vi "Parse Data Frame.vi"(0 "VISA Session In":refnum<visa-resource-name>="Alicat", 5 "Unit ID (A)":string="A", 7 "Data Frame Input":string, 9 "Data Frame Format In":T1, 11 "error in":errorcluster, 13 "Offset (2 if polling, 0 if streaming)":u32=2) -> (1 "Range Exceeded":bool, 3 "Error/Overrange/Unknown String":string, 4 "VISA Session Out":refnum<visa-resource-name>, 6 "Data Cluster":T2, 10 "Data Frame Format Out":T1, 12 "Error Present":bool, 14 "Unknown Dataframe Info":bool, 15 "error out":errorcluster)   [LabVIEW 2016]
doc: "Parses data string obtained from an Alicat device according to data flag inputs, and if none are present the device will query the data flags (adding a considerable amount of time to the VI's execution). Outputs cluster of data, retrieved/used data flags, and error/overrange/unknown indicators and strings."
uses:
  <vilib>/Utility/error.llb/whitespace.ctl
panel:
  # "Totalizer Timer"
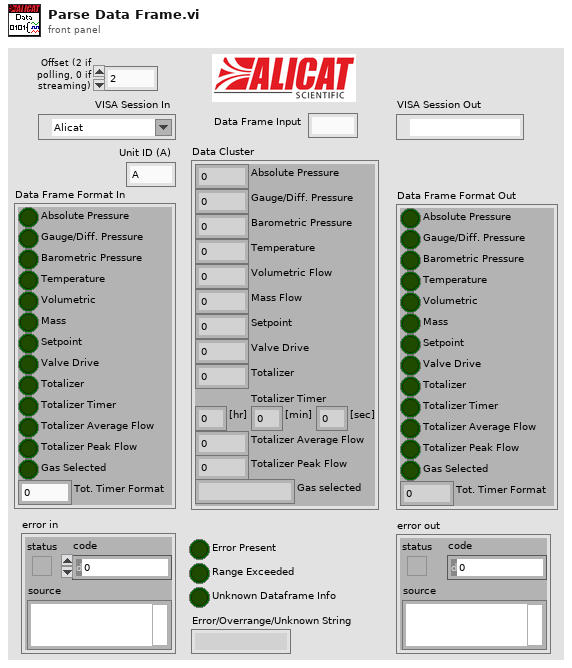
[diagram p1: front panel]
types:
  T1 = cluster{"Absolute Pressure":bool, "Gauge/Diff. Pressure":bool, "Barometric Pressure":bool, "Temperature":bool, "Volumetric":bool, "Mass":bool, "Setpoint":bool, "Valve Drive":bool, "Totalizer":bool, "Totalizer Timer":bool, "Totalizer Average Flow":bool, "Totalizer Peak Flow":bool, "Gas Selected":bool, "Tot. Timer Format":u16}
  T2 = cluster{"Absolute Pressure":dbl, "Gauge/Diff. Pressure":dbl, "Barometric Pressure":dbl, "Temperature":dbl, "Volumetric Flow":dbl, "Mass Flow":dbl, "Setpoint":dbl, "Valve Drive":dbl, "Totalizer":dbl, "[hr]":dbl, "[min]":dbl, "[sec]":dbl, "Totalizer Average Flow":dbl, "Totalizer Peak Flow":dbl, "Gas selected":string}
  T3 = cluster{"Absolute Pressure":dbl, "Gauge/Diff. Pressure":dbl, "Barometric Pressure":dbl, "Temperature":dbl, "Volumetric":dbl, "Mass":dbl, "Setpoint":dbl, "Valve Drive":dbl, "Totalizer":dbl, "[hr]":dbl, "[min]":dbl, "[sec]":dbl, "Totalizer Average Flow":dbl, "Totalizer Peak Flow":dbl, "Gas selected":string}
  T4 = typedef "whitespace.ctl" = u16
  T5 = cluster{"Absolute Pressure":bool, "Gauge/Diff. Pressure":bool, "Barometric Pressure":bool, "Temperature":bool, "Volumetric":bool, "Mass":bool, "Setpoint":bool, "Valve Drive":bool, "Totalizer":bool, "Totalizer Timer":bool, "Totalizer Average Flow":bool, "Totalizer Peak Flow":bool, "Gas Selected":bool}
  T6 = cluster{"[0]":dbl, "[1]":dbl, "[2]":dbl, "[3]":dbl, "[4]":dbl, "[5]":dbl, "[6]":dbl, "[7]":dbl, "[8]":dbl, "[9]":dbl, "[10]":dbl, "[11]":dbl}
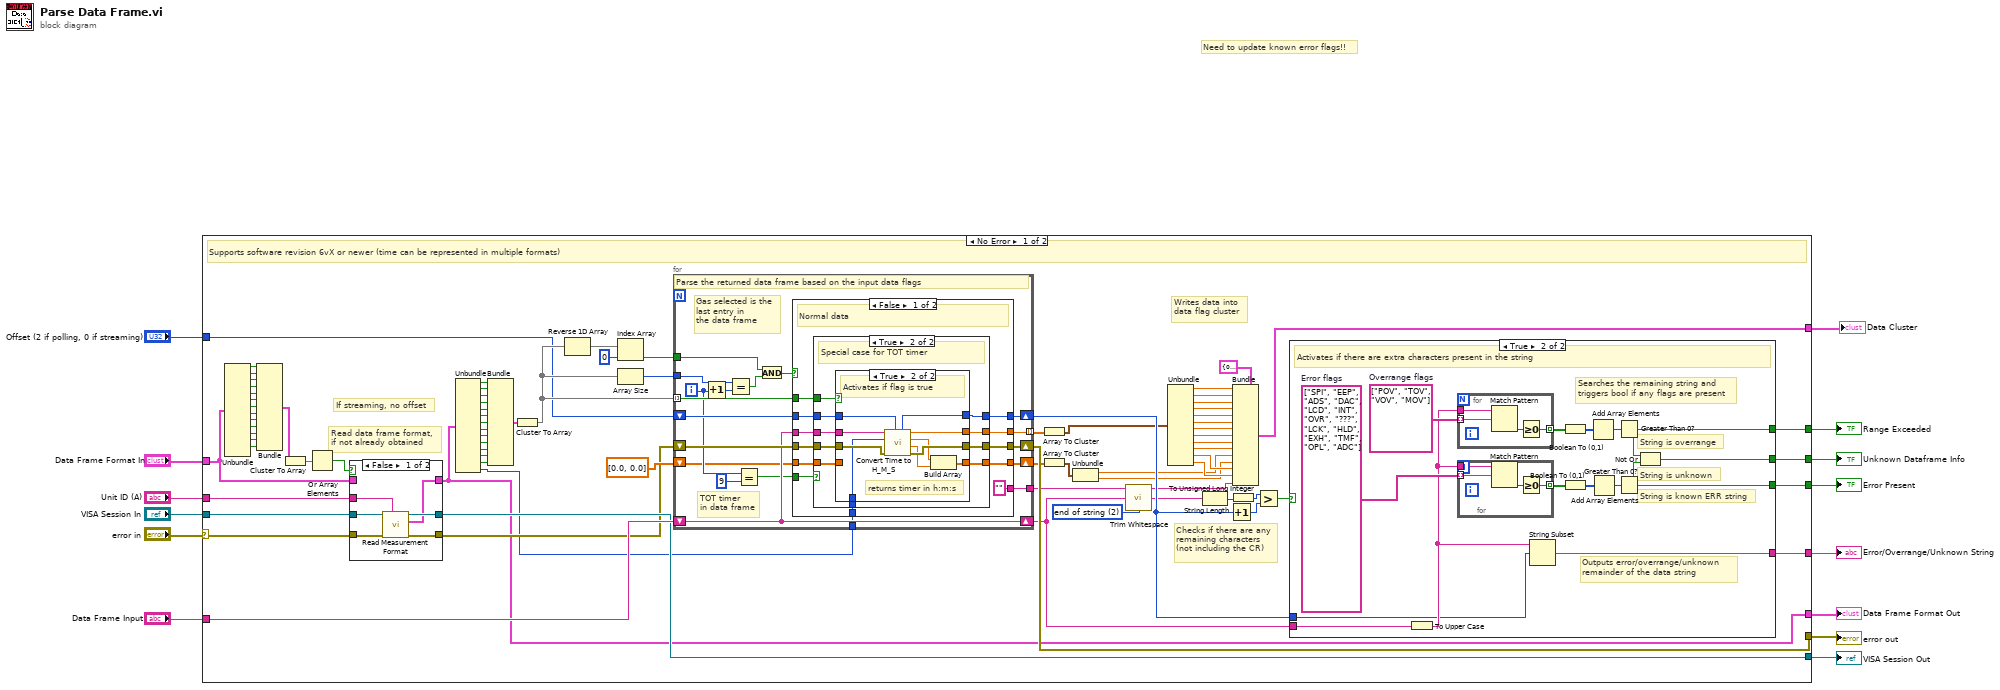
[diagram p0: block diagram]
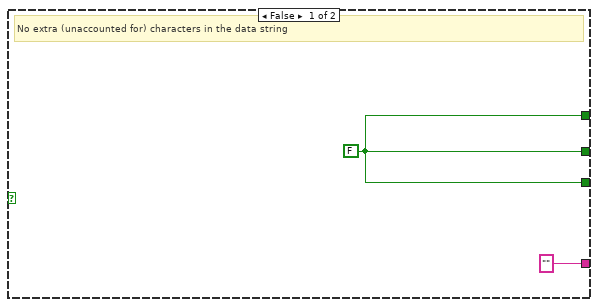
[diagram p2: hidden frame]
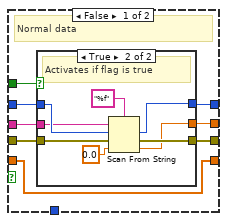
[diagram p3: hidden frame]
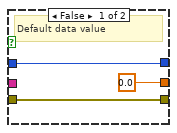
[diagram p4: hidden frame]
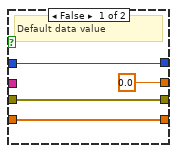
[diagram p5: hidden frame]
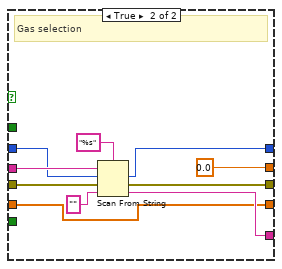
[diagram p6: hidden frame]
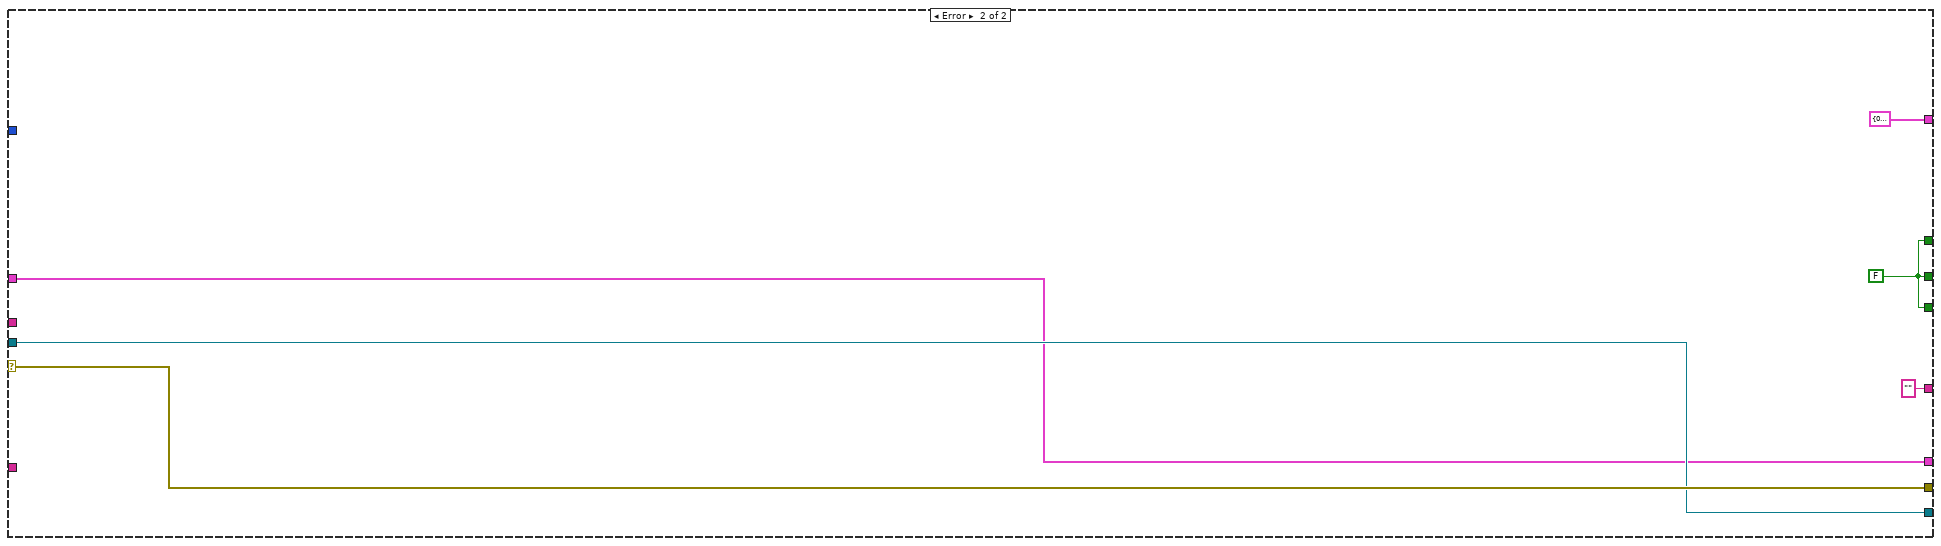
[diagram p8: hidden frame]
diagram:
  # "Need to update known error flags!!"
  n1 = case shown="No Error" "error in" {
    selector: "error in" -> [w50 w218]
    tunnel: "VISA Session In" -> [w94 w217]
    tunnel: "Unit ID (A)" -> [w93 _]
    tunnel: [w92 w214] -> w12
    tunnel: [w91 w214] -> w11
    tunnel: [w90 w214] -> w10
    tunnel: [w89 ""] -> w9
    tunnel: [w48 w217] -> w8
    tunnel: [w88 w218] -> w7
    tunnel: "Data Frame Format In" -> [w31 w216]
    tunnel: [w16 w216] -> w5
    tunnel: [w87 T3 {"Absolute Pressure"=0.0, "Gauge/Diff. Pressure"=0.0, "Barometric Pressure"=0.0, "Temperature"=0.0, "Volumetric"=0.0, "Mass"=0.0, "Setpoint"=0.0, "Valve Drive"=0.0, "Totalizer"=0.0, "[hr]"=0.0, "[min]"=0.0, "[sec]"=0.0, "Totalizer Average Flow"=0.0, "Totalizer Peak Flow"=0.0, "Gas selected"=""} ("Data Cluster 2")] -> w4
    tunnel: "Data Frame Input" -> [w49 _]
    tunnel: "Offset (2 if polling, 0 if streaming)" -> [w46 _]
    frame No Error {
      w62 = T4 2 items=["both", "start of string", "end of string"] ("location (both)")
      # "If streaming, no offset"
      # "Checks if there are any\nremaining characters\n(not including the CR)"
      # "Writes data into \ndata flag cluster"
      # "Read data frame format, \nif not already obtained"
      # "Supports software revision 6vX or newer (time can be represented in multiple formats)"
      n2 = Unbundle(w31) -> ("Absolute Pressure"=w45:bool, "Gauge/Diff. Pressure"=w33:bool, "Barometric Pressure"=w34:bool, "Temperature"=w35:bool, "Volumetric"=w36:bool, "Mass"=w37:bool, "Setpoint"=w38:bool, "Valve Drive"=w39:bool, "Totalizer"=w40:bool, "Totalizer Timer"=w41:bool, "Totalizer Average Flow"=w42:bool, "Totalizer Peak Flow"=w43:bool, "Gas Selected"=w44:bool)  [unwired: 1 out]
      n3 = Bundle("Absolute Pressure"=w45, "Gauge/Diff. Pressure"=w33, "Barometric Pressure"=w34, "Temperature"=w35, "Volumetric"=w36, "Mass"=w37, "Setpoint"=w38, "Valve Drive"=w39, "Totalizer"=w40, "Totalizer Timer"=w41, "Totalizer Average Flow"=w42, "Totalizer Peak Flow"=w43, "Gas Selected"=w44) -> (w32:T5)  [unwired: 1 in]
      n4 = Cluster To Array(cluster=w32) -> (array=w86:bool[])
      n5 = Or Array Elements(Boolean array=w86) -> (logical OR=w85:bool)
      n6 = case shown="False" w85 {
        tunnel: [w205 w210] -> w16
        tunnel: w94 -> [w209 w212]
        tunnel: w50 -> [w208 w211]
        tunnel: [w207 w212] -> w48
        tunnel: [w206 w211] -> w47
        tunnel: w31 -> [_ w210]
        tunnel: w93 -> [w204 _]
        frame False {
          n7 = call "Read Measurement Format.vi"("Unit ID (A)"=w204, "error in"=w208, "VISA Session In"=w209) -> ("error out"=w206:errorcluster, "Data Frame Format"=w205:T1, "VISA Session Out"=w207:refnum<visa-resource-name>)  [unwired: 6 in]
        }
        frame True {
        }
      }
      n8 = Unbundle(w16) -> ("Absolute Pressure"=w30:bool, "Gauge/Diff. Pressure"=w18:bool, "Barometric Pressure"=w19:bool, "Temperature"=w20:bool, "Volumetric"=w21:bool, "Mass"=w22:bool, "Setpoint"=w23:bool, "Valve Drive"=w24:bool, "Totalizer"=w25:bool, "Totalizer Timer"=w26:bool, "Totalizer Average Flow"=w27:bool, "Totalizer Peak Flow"=w28:bool, "Gas Selected"=w29:bool, "Tot. Timer Format"=w15:u16)
      n9 = Bundle("Absolute Pressure"=w30, "Gauge/Diff. Pressure"=w18, "Barometric Pressure"=w19, "Temperature"=w20, "Volumetric"=w21, "Mass"=w22, "Setpoint"=w23, "Valve Drive"=w24, "Totalizer"=w25, "Totalizer Timer"=w26, "Totalizer Average Flow"=w27, "Totalizer Peak Flow"=w28, "Gas Selected"=w29) -> (w17:T5)  [unwired: 1 in]
      n10 = Cluster To Array(cluster=w17) -> (array=w66:bool[])
      n11 = Reverse 1D Array(array=w66) -> (reversed array=w65:bool[])
      n12 = Index Array(array=w65, index=0) -> (element=w63:bool)
      n13 = Array Size(array=w66) -> (size(s)=w75:i32)
      n14 = for {
        shift-right: [w133] -> w61
        shift-left: w49 -> [w133]
        tunnel: w66 -> [w132] mode=indexing
        shift-right: [w136] -> w71
        shift-left: w46 -> [w138]
        shift-right: [w135] -> w88
        shift-left: w47 -> [w137]
        tunnel: [w134] -> w84 mode=indexing
        tunnel: [w131] -> w57
        tunnel: w75 -> [w130]
        shift-right: [w125] -> w68
        shift-left: dbl[] [0.0, 0.0] -> [w124]
        tunnel: w63 -> [w121]
        tunnel: w15 -> [w120]
        i -> [w127]
        # "TOT timer \nin data frame"
        # "Gas selected is the \nlast entry in\nthe data frame"
        # "Parse the returned data frame based on the input data flags"
        n15 = Increment(x=w127) -> (x+1=w129:i32)
        n16 = Equal?(x=w130, y=w129) -> (x = y?=w123:bool)
        n17 = Equal?(x=w127, y=9) -> (x = y?=w128:bool)
        n18 = And(x=w121, y=w123) -> (x .and. y?=w122:bool)
        n19 = case shown="False" w122 {
          tunnel: w138 -> [w150 w197]
          tunnel: w137 -> [w149 w200]
          tunnel: [w148 w203] -> w136
          tunnel: [w147 w202] -> w135
          tunnel: [w146 0.0 ("default value 1")] -> w134
          tunnel: w133 -> [w145 w201]
          tunnel: w132 -> [w144 _]
          tunnel: ["" ("default value 1") w198] -> w131
          tunnel: w128 -> [w142 _]
          tunnel: [w141 w196] -> w125
          tunnel: w124 -> [w140 w196]
          tunnel: w120 -> [w139 _]
          frame False {
            # "Normal data"
            n20 = case shown="True" w142 {
              tunnel: w150 -> [w158 w174]
              tunnel: w149 -> [w157 w176]
              tunnel: [w156 w179] -> w148
              tunnel: [w155 w177] -> w147
              tunnel: [w154 w178] -> w146
              tunnel: w145 -> [w153 w175]
              tunnel: w144 -> [w152 w173]
              tunnel: [w151 w172] -> w141
              tunnel: w140 -> [w151 w171]
              tunnel: w139 -> [_ w170]
              frame False {
                # "Normal data"
                n21 = case shown="True" w152 {
                  tunnel: w158 -> [w159 w169]
                  tunnel: w153 -> [_ w168]
                  tunnel: w157 -> [w160 w167]
                  tunnel: [w159 w166] -> w156
                  tunnel: [w160 w165] -> w155
                  tunnel: [0.0 ("default value 1") w162] -> w154
                  frame False {
                    # "Default data value"
                  }
                  frame True {
                    # "Activates if flag is true"
                    n22 = Scan From String(format string="%f", input string=w168, initial scan location=w169, error in=w167, default 1=0.0 ("default value 1")) -> (offset past scan=w166:u32, error out=w165:errorcluster, output 1=w162:dbl)  [unwired: 1 out]
                  }
                }
              }
              frame True {
                # "Special case for TOT timer"
                n23 = case shown="True" w173 {
                  tunnel: w174 -> [w181 w192]
                  tunnel: w175 -> [_ w190]
                  tunnel: w176 -> [w182 w189]
                  tunnel: [w181 w191] -> w179
                  tunnel: [w182 w188] -> w177
                  tunnel: [0.0 ("default value 1") w186] -> w178
                  tunnel: [w180 w193] -> w172
                  tunnel: w171 -> [w180 _]
                  tunnel: w170 -> [_ w187]
                  frame False {
                    # "Default data value"
                  }
                  frame True {
                    # "returns timer in h:m:s"
                    # "Activates if flag is true"
                    n24 = call "Convert Time to H_M_S.vi"("Initial Scan Location"=w192, "error in"=w189, "Tot. Timer Format"=w187, "Time Data String"=w190) -> ("error out"=w188:errorcluster, "[sec]"=w184:dbl, "[min]"=w185:dbl, "[hr]"=w186:dbl, "Offset Past Scan"=w191:u32)  [unwired: 3 in]
                    n25 = Build Array(w185, w184) -> (w193:dbl[])
                  }
                }
              }
            }
          }
          frame True {
            # "Gas selection"
            n26 = Scan From String(format string="%s", input string=w201, initial scan location=w197, error in=w200, default 1="" ("format string")) -> (offset past scan=w203:u32, error out=w202:errorcluster, output 1=w198:string)  [unwired: 1 out]
          }
        }
      }
      n27 = Array To Cluster(array=w84) -> (cluster=w59:T6)
      n28 = Array To Cluster(array=w68) -> (cluster=w67:cluster{"[0]":dbl, "[1]":dbl})
      n29 = Unbundle(w67) -> ("[0]"=w53:dbl, "[1]"=w54:dbl)
      n30 = call <vilib>:"Trim Whitespace.vi"("string"=w61, "location (both)"=w62) -> ("trimmed string"=w60:string)
      n31 = Unbundle(w59) -> ("[0]"=w83:dbl, "[1]"=w82:dbl, "[2]"=w81:dbl, "[3]"=w80:dbl, "[4]"=w79:dbl, "[5]"=w78:dbl, "[6]"=w77:dbl, "[7]"=w76:dbl, "[8]"=w51:dbl, "[9]"=w52:dbl, "[10]"=w55:dbl, "[11]"=w56:dbl)
      n32 = String Length(string=w60) -> (length=w72:i32)
      n33 = Increment(x=w71) -> (x+1=w70:u32)
      n34 = To Unsigned Long Integer(number=w72) -> (unsigned 32bit integer=w74:u32)
      n35 = Bundle(cluster=T3 {"Absolute Pressure"=0.0, "Gauge/Diff. Pressure"=0.0, "Barometric Pressure"=0.0, "Temperature"=0.0, "Volumetric"=0.0, "Mass"=0.0, "Setpoint"=0.0, "Valve Drive"=0.0, "Totalizer"=0.0, "[hr]"=0.0, "[min]"=0.0, "[sec]"=0.0, "Totalizer Average Flow"=0.0, "Totalizer Peak Flow"=0.0, "Gas selected"=""} ("Data Cluster 2"), "Absolute Pressure"=w83, "Gauge/Diff. Pressure"=w82, "Barometric Pressure"=w81, "Temperature"=w80, "Volumetric"=w79, "Mass"=w78, "Setpoint"=w77, "Valve Drive"=w76, "Totalizer"=w51, "[hr]"=w52, "[min]"=w53, "[sec]"=w54, "Totalizer Average Flow"=w55, "Totalizer Peak Flow"=w56, "Gas selected"=w57) -> (w87:T3)
      n36 = Greater?(x=w74, y=w70) -> (0:w73:bool)
      n37 = case shown="True" w73 {
        tunnel: w61 -> [_ w108]
        tunnel: [w95 w102] -> w92
        tunnel: [w95 w101] -> w91
        tunnel: w71 -> [_ w99]
        tunnel: [w95 w98] -> w90
        tunnel: ["" w97] -> w89
        frame False {
          w95 = FALSE
          # "No extra (unaccounted for) characters in the data string"
        }
        frame True {
          w111 = string[] ["SPI", "EEP", "ADS", "DAC", "LCD", "INT", "OVR", "???", "LCK", "HLD", "EXH", "TMF", "OPL", "ADC"]  # Error flags
          w110 = string[] ["POV", "TOV", "VOV", "MOV"]  # Overrange flags
          # "String is unknown"
          # "String is known ERR string"
          # "String is overrange"
          # "Outputs error/overrange/unknown\nremainder of the data string"
          # "Searches the remaining string and\ntriggers bool if any flags are present"
          # "Activates if there are extra characters present in the string"
          n38 = To Upper Case(1:w108) -> (0:w100:string)
          n39 = for {
            tunnel: w110 -> [w118] mode=indexing
            tunnel: w100 -> [w117]
            tunnel: [w116] -> w109 mode=indexing
            n40 = Match Pattern(string=w117, regular expression=w118) -> (offset past match=w119:i32)  [unwired: 1 in, 3 out]
            n41 = Greater Or Equal To 0?(x=w119) -> (x >= 0?=w116:bool)
          }
          n42 = for {
            tunnel: w111 -> [w114] mode=indexing
            tunnel: w100 -> [w113]
            tunnel: [w112] -> w107 mode=indexing
            n43 = Match Pattern(string=w113, regular expression=w114) -> (offset past match=w115:i32)  [unwired: 1 in, 3 out]
            n44 = Greater Or Equal To 0?(x=w115) -> (x >= 0?=w112:bool)
          }
          n45 = String Subset(string=w100, offset (0)=w99) -> (substring=w97:string)  [unwired: 1 in]
          n46 = Boolean To (0,1)(Boolean=w109) -> (0, 1=w105:i16[])
          n47 = Boolean To (0,1)(Boolean=w107) -> (0, 1=w104:i16[])
          n48 = Add Array Elements(numeric array=w105) -> (sum=w106:i16)
          n49 = Add Array Elements(numeric array=w104) -> (sum=w103:i16)
          n50 = Greater Than 0?(x=w106) -> (x > 0?=w101:bool)
          n51 = Greater Than 0?(x=w103) -> (x > 0?=w102:bool)
          n52 = Not Or(1:w102, 2:w101) -> (0:w98:bool)
        }
      }
    }
    frame Error {
      w214 = FALSE
    }
  }
  "error out" <- w7
  "VISA Session Out" <- w8
  "Error Present" <- w12
  "Range Exceeded" <- w11
  "Unknown Dataframe Info" <- w10
  "Error/Overrange/Unknown String" <- w9
  "Data Cluster" <- w4
  "Data Frame Format Out" <- w5
